vi "Test LIA Filtering.vi"() -> ()   [LabVIEW 2019]
uses:
  <vilib>/measure/NI_MABase.lvlib
  <vilib>/Analysis/NI_AALBase.lvlib
  src/DSP/DSP.lvclass
  src/Instrument.Lockin/Instrument.Lockin.lvclass
  src/Instrument.DAQ/Typedefs/REF.Channel--Cluster.ctl
  src/Instrument.DAQ/Instrument.DAQ.lvclass
  <vilib>/Analysis/baseanly.llb/Mean (DBL).vi
panel:
  out "order (n)":i32
  out "Time constant (s)":dbl
  out "Waveform Graph":waveform(dbl)[](graph)
  out "XY Graph 2":cluster{i32[], dbl[]}[](graph)
  out "elapsed":dbl
  out "Decimating":i32
  out "Fs":dbl
  out "XY Graph":cluster{"Fs":dbl[], dbl[]}[](graph)
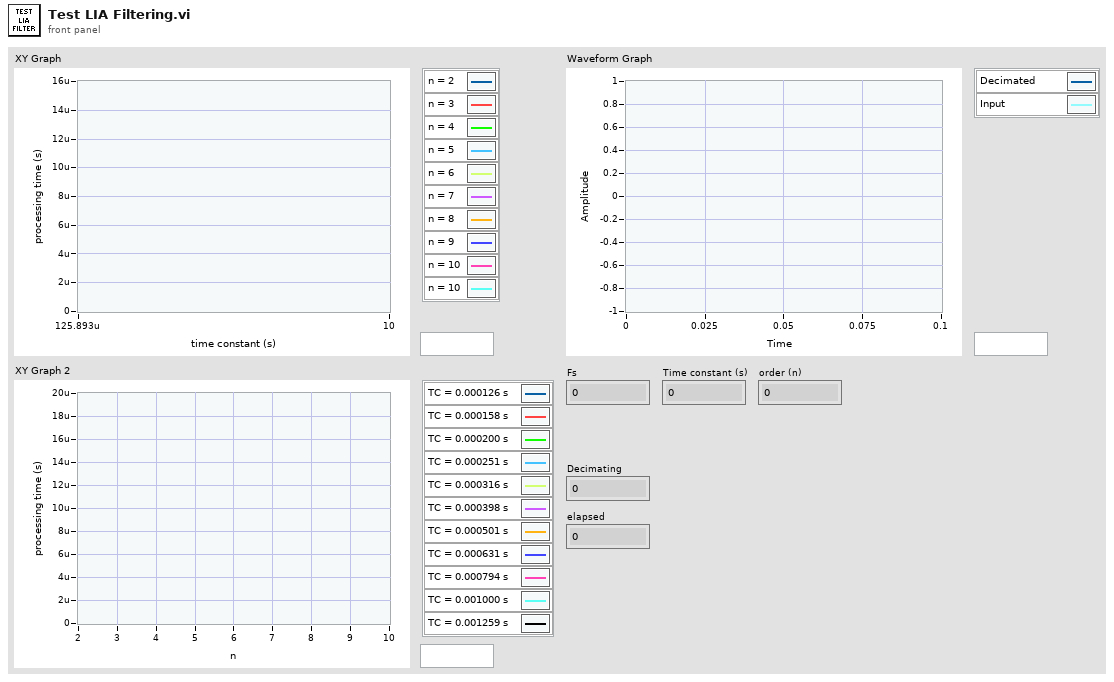
[diagram p1: front panel]
types:
  T1 = typedef "Instrument.Lockin.lvlib/Instrument.DAQ.lvclass/REF.Channel--Cluster.ctl" = cluster{"Enable?":bool, "Channel":i32, "Frequency":dbl, "Phase":dbl, "TC":dbl, "Roll-Off":i32}
  T2 = cluster{"Fs.Output (S/s)":dbl, "Decimation Factor":i32, "Settling Time (s)":dbl, "Noise Bandwidth (Hz)":dbl, "-3dB Bandwidth (Hz)":dbl, "Attenuation (dB)":dbl}
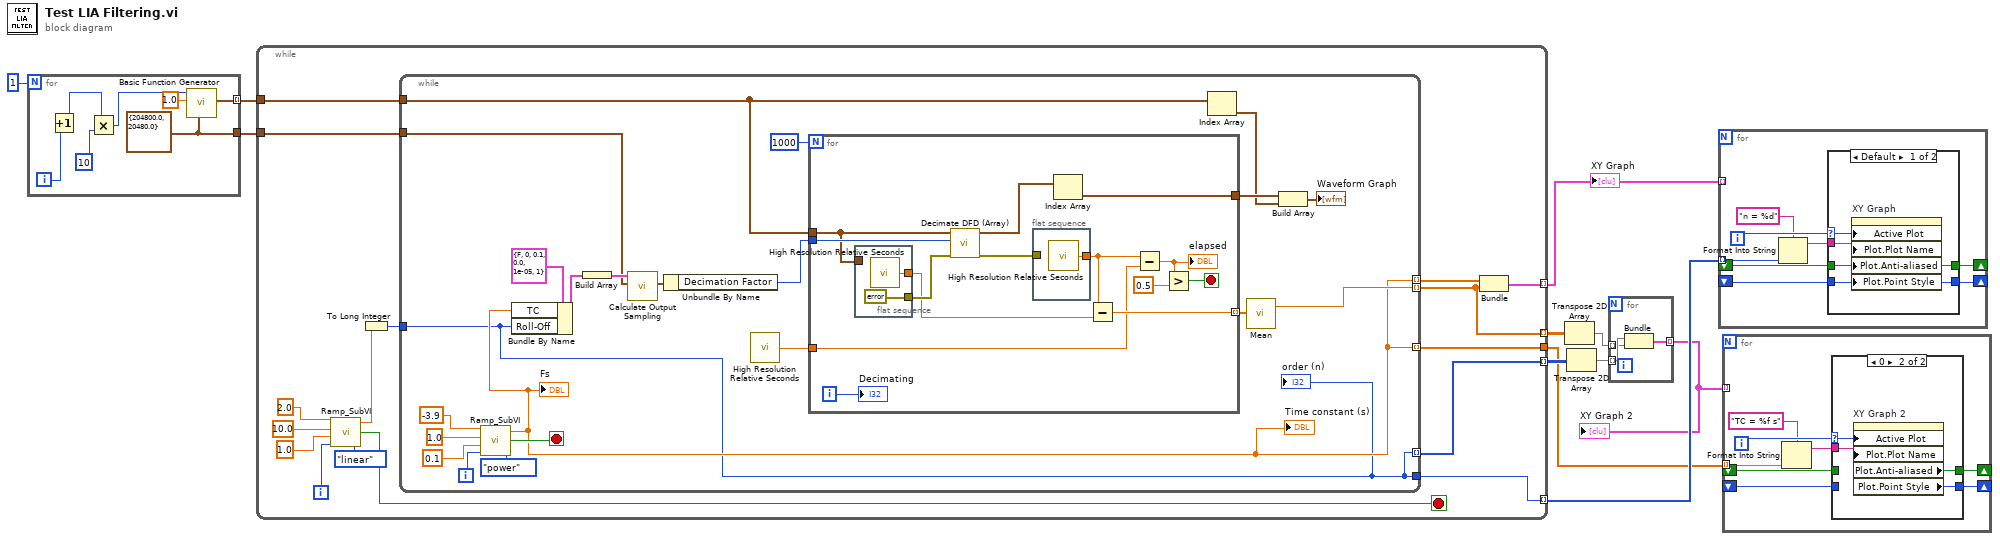
[diagram p0: block diagram]
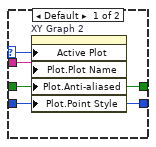
[diagram p2: hidden frame]
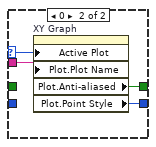
[diagram p3: hidden frame]
diagram:
  n1 = for {
    N: 1 -> [_]
    tunnel: [w18] -> w9 mode=indexing
    tunnel: [w16] -> w10
    i -> [w17]
    w16 = cluster{"Fs":dbl, "#s":dbl} {"Fs"=204800.0, "#s"=20480.0} ("sampling info")
    n2 = Increment(x=w17) -> (x+1=w13:i32)
    n3 = Multiply(x=w13, y=10) -> (x*y=w12:i32)
    n4 = call <vilib>:"Basic Function Generator.vi"("sampling info"=w16, "amplitude"=1.0, "frequency"=w12) -> ("signal out"=w18:waveform(dbl))  [unwired: 6 in, 2 out]
  }
  n5 = while {
    tunnel: w10 -> [w34]
    tunnel: w9 -> [w33]
    tunnel: [w24] -> w8 mode=indexing
    tunnel: [w19] -> w7 mode=indexing
    tunnel: [w22] -> w6 mode=indexing
    tunnel: [w21] -> w5 mode=indexing
    tunnel: [w20] -> w1
    i -> [w29]
    stop <- w27 stop-if-true
    n6 = call <userlib>:"Ramp_SubVI.vi"("Enum"=enum16{"linear", "power"}."linear", "index"=w29, "step"=1.0, "end"=10.0, "start"=2.0) -> ("Stop?"=w27:bool, "Numeric"=w28:dbl)
    n7 = To Long Integer(number=w28) -> (32bit integer=w23:i32)
    n8 = while {
      tunnel: w33 -> [w48]
      tunnel: w34 -> [w43]
      tunnel: [w38] -> w25 mode=indexing
      tunnel: [w39] -> w22 mode=indexing
      tunnel: w23 -> [w37]
      tunnel: [w37] -> w21 mode=indexing
      tunnel: [w38] -> w20 mode=indexing
      tunnel: [w37] -> w19
      i -> [w56]
      stop <- w49 stop-if-true
      (unwired) 0
      n9 = call <userlib>:"Ramp_SubVI.vi"("Enum"=enum16{"linear", "power"}."power", "index"=w56, "step"=0.1, "end"=1.0, "start"=-3.9) -> ("Stop?"=w49:bool, "Numeric"=w38:dbl)
      "Fs" <- w38
      "Time constant (s)" <- w38
      n10 = Bundle By Name(cluster=T1 {"Enable?"=FALSE, "Channel"=0, "Frequency"=0.1, "Phase"=0.0, "TC"=1e-05, "Roll-Off"=1} ("REF"), "TC"=w38, "Roll-Off"=w37) -> (w46:T1)
      n11 = Build Array(w46) -> (w45:T1[])
      n12 = call "Calculate Output Sampling.vi"("sampling info"=w43, "Cfg_REF"=w45) -> ("Filter Parameters"=w36:T2)  [unwired: 8 in, 1 out]
      n13 = Unbundle By Name(w36) -> ("Decimation Factor"=w35:i32)
      n14 = call <vilib>:"High Resolution Relative Seconds.vi"() -> ("relative seconds"=w40:dbl)
      n15 = for {
        N: 1000 -> [_]
        tunnel: w35 -> [w70]
        tunnel: w48 -> [w57]
        tunnel: [w62] -> w41 mode=indexing
        tunnel: w40 -> [w60]
        tunnel: [w58] -> w51
        i -> [w66]
        stop <- w68 stop-if-true
        n16 = flat-sequence {
          tunnel: [w72] -> w63
          tunnel: w57 -> [_]
          tunnel: [errorcluster {"status"=FALSE, "code"=0, "source"=""} ("error in (no error)")] -> w64
          frame #0 {
            n17 = call <vilib>:"High Resolution Relative Seconds.vi"() -> ("relative seconds"=w72:dbl)
          }
        }
        n18 = call "Decimate DFD (Array).vi"("error in (no error)"=w64, "Decimation Factor"=w70, "Waveforms in"=w57) -> ("error out"=w65:errorcluster, "waveforms out"=w59:waveform(dbl)[])  [unwired: 7 in]
        n19 = flat-sequence {
          tunnel: [w73] -> w61
          tunnel: w65 -> [_]
          frame #0 {
            n20 = call <vilib>:"High Resolution Relative Seconds.vi"() -> ("relative seconds"=w73:dbl)
          }
        }
        n21 = Index Array(array=w59) -> (element=w58:waveform(dbl))  [unwired: 1 in]
        n22 = Subtract(x=w61, y=w63) -> (x-y=w62:dbl)
        n23 = Subtract(x=w61, y=w60) -> (x-y=w69:dbl)
        "elapsed" <- w69
        n24 = Greater?(x=w69, y=0.5) -> (0:w68:bool)
        "Decimating" <- w66
      }
      n25 = Index Array(array=w48) -> (element=w50:waveform(dbl))  [unwired: 1 in]
      n26 = call-poly <vilib>:"Mean.vi"("X"=w41) -> ("mean"=w39:dbl)  [unwired: 1 out]
      n27 = Build Array(w51, w50) -> (→"Waveform Graph":waveform(dbl)[])
      "order (n)" <- w37
    }
    n28 = Bundle(w25, w22) -> (w24:cluster{dbl[], dbl[]})  [unwired: 1 in]
  }
  "XY Graph" <- w8
  n29 = Transpose 2D Array(2D array=w6) -> (transposed array=w3:dbl[][])
  n30 = Transpose 2D Array(2D array=w5) -> (transposed array=w4:i32[][])
  n31 = for {
    tunnel: w4 -> [w76] mode=indexing
    tunnel: w3 -> [w75] mode=indexing
    tunnel: [w74] -> w2 mode=indexing
    n32 = Bundle(w76, w75) -> (w74:cluster{i32[], dbl[]})  [unwired: 1 in]
  }
  "XY Graph 2" <- w2
  n33 = for {
    tunnel: w7 -> [w83] mode=indexing
    shift-right: [w80] -> _
    shift-left: _ -> [w78]
    shift-right: [w79] -> _
    shift-left: _ -> [w77]
    tunnel: w8 -> [_] mode=indexing
    i -> [w84]
    n34 = Format Into String(format string="n = %d", w83) -> (resulting string=w81:string)  [unwired: 2 in, 1 out]
    n35 = case shown="Default" w84 {
      selector: w84 -> [w88 w92]
      tunnel: w81 -> [w87 w91]
      tunnel: [w86 w90] -> w80
      tunnel: [w85 w89] -> w79
      tunnel: w78 -> [w86 _]
      tunnel: w77 -> [w85 _]
      frame Default {
        n36 = property on="XY Graph" class="XYGraph (strict)"("Active Plot"=w88, "Plot.Plot Name"=w87, "Plot.Anti-aliased"=w86, "Plot.Point Style"=w85) -> ()  [unwired: 2 in, 2 out]
      }
      frame 0 {
        n37 = property on="XY Graph" class="XYGraph (strict)"("Active Plot"=w92, "Plot.Plot Name"=w91) -> ("Plot.Anti-aliased"=w90:bool, "Plot.Point Style"=w89:u8)  [unwired: 2 in, 2 out]
      }
    }
  }
  n38 = for {
    tunnel: w1 -> [w99] mode=indexing
    shift-right: [w96] -> _
    shift-left: _ -> [w94]
    shift-right: [w95] -> _
    shift-left: _ -> [w93]
    tunnel: w2 -> [_] mode=indexing
    i -> [w100]
    n39 = Format Into String(format string="TC = %f s", w99) -> (resulting string=w97:string)  [unwired: 2 in, 1 out]
    n40 = case shown="0" w100 {
      selector: w100 -> [w104 w108]
      tunnel: w97 -> [w103 w107]
      tunnel: [w102 w106] -> w96
      tunnel: [w101 w105] -> w95
      tunnel: w94 -> [w102 _]
      tunnel: w93 -> [w101 _]
      frame Default {
        n41 = property on="XY Graph 2" class="XYGraph (strict)"("Active Plot"=w104, "Plot.Plot Name"=w103, "Plot.Anti-aliased"=w102, "Plot.Point Style"=w101) -> ()  [unwired: 2 in, 2 out]
      }
      frame 0 {
        n42 = property on="XY Graph 2" class="XYGraph (strict)"("Active Plot"=w108, "Plot.Plot Name"=w107) -> ("Plot.Anti-aliased"=w106:bool, "Plot.Point Style"=w105:u8)  [unwired: 2 in, 2 out]
      }
    }
  }
